vi "Show Peaks & Valleys.vi"(6 "peaksValleysOptions":T1={"Peaks"={"#"=2, "size"=0, "WidthThreshold"=2, "AmplitudeThreshold"=2.0, "Fill"=FALSE, "PlotIndexes (All)"=[]}, "Valleys"={"#"=0, "size"=2, "WidthThreshold"=2, "AmplitudeThreshold"=2.0, "Fill"=FALSE, "PlotIndexes (All)"=[]}} {"Valleys"."AmplitudeThreshold" min=0.0 format="%.3f"; "Valleys"."WidthThreshold" min=3; "Valleys"."size" min=1 max=50; "Peaks"."AmplitudeThreshold" min=0.0 format="%.3f"; "Peaks"."WidthThreshold" min=3; "Peaks"."size" min=1 max=50}, 8 "error in (no error)":errorcluster, 10 "XY Graph":refnum<vi>, 11 "input picture":picture) -> (0 "error out":errorcluster, 3 "output picture":picture)   [LabVIEW 2014, in "Graph Extensions.lvlib"]
doc: "Peaks and Valleys can be set on a per plot basis, with individual settings. \n\n<B>#</b> - Defines how many peaks or valleys to show. For peaks, they are shown in descending amplitude, so the highest peaks first. For valleys, they are shown in ascending amplitude, so the lower valleys first.\n<b>size</b> - How many pixels large is the peak or valley icon shown in the overlay.\n<b>widthThreshold</b> - Sets the X axis width range used to identify a peak or valley within. Only a single peak can be identified within this Xaxis width, so the wider it is, the less peaks you will find. This is needed to help filter out noise or minor up and downs, which are not true peaks in the data set.\n<b>AmplitudeThreshold</b> - Sets the Y axis range that is required to identify a peak or valley from. This as well helps filter out noise and identify the minimum amplitude that a peak or valley must have above or below its neighbors in th width threshold range.\n<b>PlotIndexes</b> - By default, all plots are used, but you can limit the peak or valley to an array of individual plot numbers."
uses:
  Graph Extensions.lvlib
  controls/PeaksValleyOptions.ctl
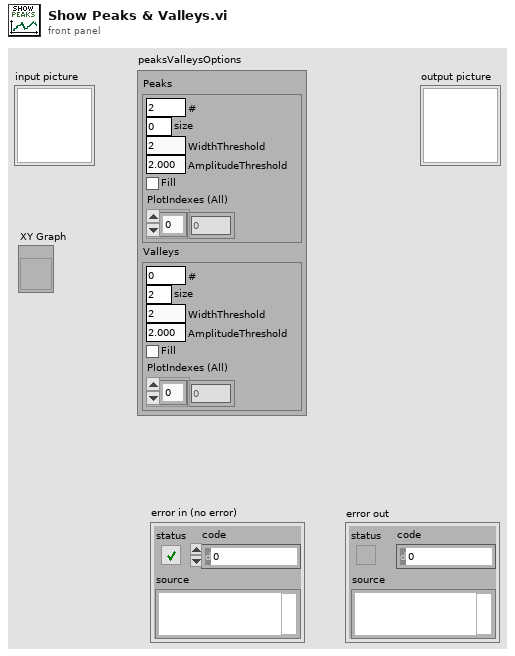
[diagram p1: front panel]
types:
  T1 = typedef "Graph Extensions.lvlib/PeaksValleyOptions.ctl" = cluster{"Peaks":cluster{"#":i32, "size":i16, "WidthThreshold":i32, "AmplitudeThreshold":dbl, "Fill":bool, "PlotIndexes (All)":u16[]}, "Valleys":cluster{"#":i32, "size":i16, "WidthThreshold":i32, "AmplitudeThreshold":dbl, "Fill":bool, "PlotIndexes (All)":u16[]}}
  T2 = cluster{"#":i32, "size":i16, "WidthThreshold":i32, "AmplitudeThreshold":dbl, "Fill":bool, "PlotIndexes (All)":u16[]}
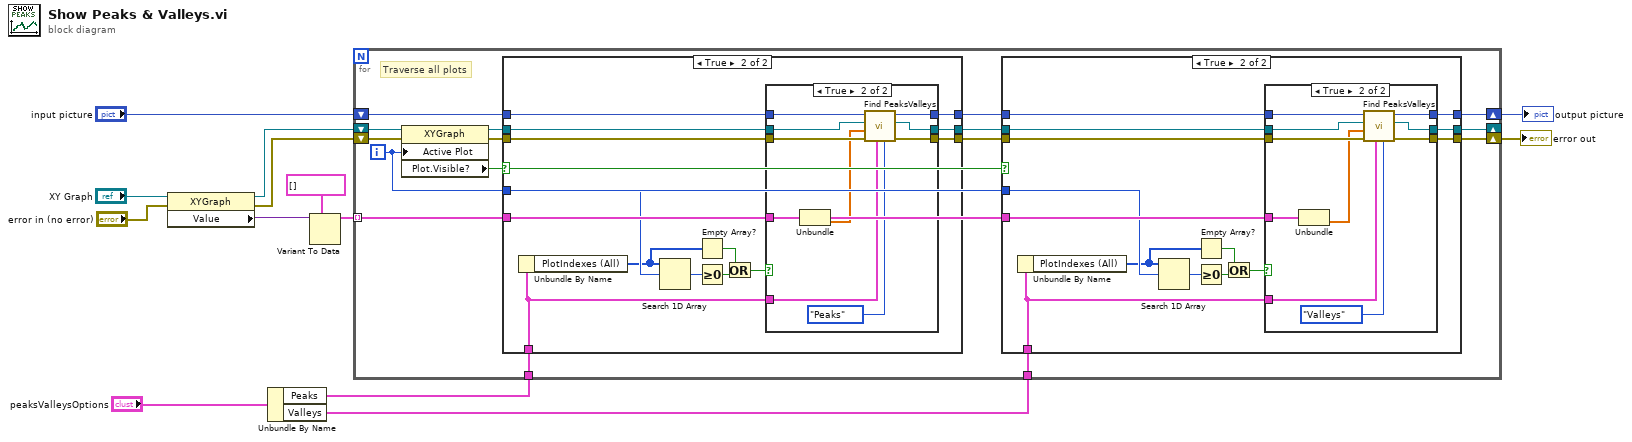
[diagram p0: block diagram]
diagram:
  n1 = property class="XYGraph"(reference="XY Graph", error in="error in (no error)") -> (reference out=w5:refnum<vi>, error out=w3:errorcluster, "Value"=w6:variant)
  n2 = Unbundle By Name("peaksValleysOptions") -> ("Peaks"=w1:T2, "Valleys"=w2:T2)
  n3 = Variant To Data(type=cluster{dbl[], dbl[]}[] [], Variant=w6) -> (data=w8:cluster{dbl[], dbl[]}[])  [unwired: 1 in, 1 out]
  n4 = for {
    tunnel: w8 -> [w14] mode=indexing
    shift-right: [w19] -> _
    shift-left: w5 -> [w28]
    shift-right: [w20] -> w11
    shift-left: "input picture" -> [w29]
    shift-right: [w18] -> w13
    shift-left: w3 -> [w26]
    tunnel: w2 -> [w17]
    tunnel: w1 -> [w24]
    i -> [w15]
    # "Traverse all plots"
    n5 = property on="Property Node" class="XYGraph"(reference=w28, error in=w26, "Active Plot"=w15) -> (reference out=w27:refnum<vi>, error out=w25:errorcluster, "Plot.Visible?"=w16:bool)
    n6 = case shown="True" w16 {
      tunnel: [w62 w70] -> w22
      tunnel: w14 -> [_ w76]
      tunnel: w29 -> [w61 w73]
      tunnel: w27 -> [w62 w71]
      tunnel: [w61 w72] -> w23
      tunnel: w25 -> [w60 w75]
      tunnel: [w60 w74] -> w21
      tunnel: w24 -> [_ w69]
      tunnel: w15 -> [_ w68]
      frame False {
        # "plot is not visible, so don't show the cursor for it."
      }
      frame True {
        n7 = Unbundle By Name(w69) -> ("PlotIndexes (All)"=w66:u16[])
        n8 = Search 1D Array(1D array=w66, element=w68) -> (index of element=w67:i32)  [unwired: 1 in]
        n9 = Empty Array?(array=w66) -> (empty?=w64:bool)
        n10 = Greater Or Equal To 0?(x=w67) -> (x >= 0?=w65:bool)
        n11 = Or(x=w64, y=w65) -> (x .or. y?=w63:bool)
        n12 = case shown="True" w63 {
          tunnel: w76 -> [_ w89]
          tunnel: w75 -> [w77 w88]
          tunnel: [w77 w87] -> w74
          tunnel: w73 -> [w79 w86]
          tunnel: [w79 w85] -> w72
          tunnel: w71 -> [w78 w84]
          tunnel: [w78 w83] -> w70
          tunnel: w69 -> [_ w81]
          frame False {
          }
          frame True {
            n13 = Unbundle(w89) -> (w80:dbl[])  [unwired: 1 out]
            n14 = call "Find PeaksValleys.vi"("peaks/valleys"=enum32{"Peaks", "Valleys"}."Peaks", "Options"=w81, "error in (no error)"=w88, "Data Array"=w80, "XYGraph in"=w84, "input picture in"=w86) -> ("error out"=w87:errorcluster, "XYGraph out"=w83:refnum<vi>, "input picture out"=w85:picture)  [unwired: 3 in]
          }
        }
      }
    }
    n15 = case shown="True" w16 {
      tunnel: [w32 w40] -> w19
      tunnel: w14 -> [_ w46]
      tunnel: w23 -> [w31 w43]
      tunnel: w22 -> [w32 w41]
      tunnel: [w31 w42] -> w20
      tunnel: w21 -> [w30 w45]
      tunnel: [w30 w44] -> w18
      tunnel: w17 -> [_ w39]
      tunnel: w15 -> [_ w38]
      frame False {
        # "plot is not visible, so don't show the cursor for it."
      }
      frame True {
        n16 = Unbundle By Name(w39) -> ("PlotIndexes (All)"=w36:u16[])
        n17 = Search 1D Array(1D array=w36, element=w38) -> (index of element=w37:i32)  [unwired: 1 in]
        n18 = Empty Array?(array=w36) -> (empty?=w34:bool)
        n19 = Greater Or Equal To 0?(x=w37) -> (x >= 0?=w35:bool)
        n20 = Or(x=w34, y=w35) -> (x .or. y?=w33:bool)
        n21 = case shown="True" w33 {
          tunnel: w46 -> [_ w59]
          tunnel: w45 -> [w47 w58]
          tunnel: [w47 w57] -> w44
          tunnel: w43 -> [w49 w56]
          tunnel: [w49 w55] -> w42
          tunnel: w41 -> [w48 w54]
          tunnel: [w48 w53] -> w40
          tunnel: w39 -> [_ w51]
          frame False {
          }
          frame True {
            n22 = Unbundle(w59) -> (w50:dbl[])  [unwired: 1 out]
            n23 = call "Find PeaksValleys.vi"("peaks/valleys"=enum32{"Peaks", "Valleys"}."Valleys", "Options"=w51, "error in (no error)"=w58, "Data Array"=w50, "XYGraph in"=w54, "input picture in"=w56) -> ("error out"=w57:errorcluster, "XYGraph out"=w53:refnum<vi>, "input picture out"=w55:picture)  [unwired: 3 in]
          }
        }
      }
    }
  }
  "error out" <- w13
  "output picture" <- w11
